vi "GetColorStatus.vi"(11 "Status":T1) -> (3 "Numeric":u32)   [LabVIEW 2013]
uses:
  Device Drivers/TRAServer/StatusTRA_TypDef.ctl
  Device Drivers/TRAServer/TRAServer.lvclass
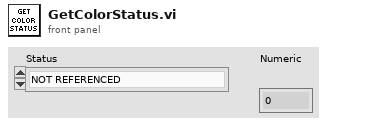
[diagram p1: front panel]
types:
  T1 = typedef "TRAServer.lvclass/StatusTRA_TypDef.ctl" = enum16{"NOT REFERENCED", "CONFIGURATION", "HOMING", "MOVING", "READY", "DISABLE", "JOGGING"}
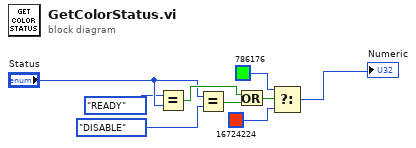
[diagram p0: block diagram]
diagram:
  n1 = Equal?(x=StatusTRA_TypDef."READY" ("y"), y="Status") -> (x = y?=w5:bool)
  n2 = Equal?(x="Status", y=StatusTRA_TypDef."DISABLE") -> (x = y?=w4:bool)
  n3 = Or(x=w5, y=w4) -> (x .or. y?=w6:bool)
  n4 = Select(t=u32 786176, s=w6, f=u32 16724224) -> (s? t:f=→"Numeric":u32)
